vi "Read Job Name.vi"(8 "error in (no error)":errorcluster, 11 "Cron.Jenkins in":refnum<class "Cron.Jenkins.lvclass">) -> (0 "error out":errorcluster, 2 "Job Name":string, 3 "Cron.Jenkins out":refnum<class "Cron.Jenkins.lvclass">)   [LabVIEW 2013, in "openCron.lvlib" / "Cron.Jenkins.lvclass"]
uses:
  Cron.Jenkins.lvclass
  Cron.Jenkins.lvclass/Cron.Jenkins.ctl
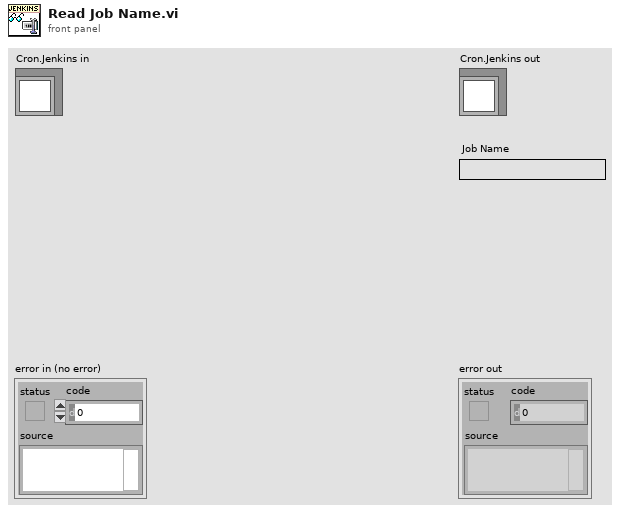
[diagram p1: front panel]
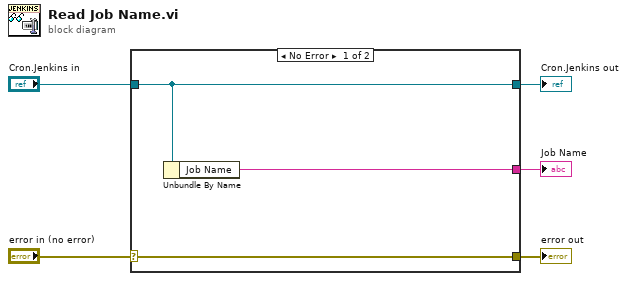
[diagram p0: block diagram]
diagram:
  n1 = case shown="No Error" "error in (no error)" {
    selector: "error in (no error)" -> [w8 w9]
    tunnel: [w8 w9] -> w4
    tunnel: [w7 w10] -> w2
    tunnel: "Cron.Jenkins in" -> [w7 w10]
    tunnel: [w6 _] -> w1
    frame No Error {
      n2 = Unbundle By Name(w7) -> ("Job Name"=w6:string)
    }
    frame Error {
    }
  }
  "error out" <- w4
  "Cron.Jenkins out" <- w2
  "Job Name" <- w1
